vi "Input Entry Init.vi"(8 "Input Control":T2, 9 "Project In":refnum<class "Project.lvclass">, 11 "Refnums":T1) -> (3 "Input Control out":refnum<vi>)   [LabVIEW 2015, in "CallVIStep.lvclass"]
uses:
  CallVIStep.lvclass
  VI Input Control Typedef.ctl
  VI Input Type Typedef.ctl
  Project.lvclass
  <vilib>/Utility/miscctls.llb/LVPointTypeDef.ctl
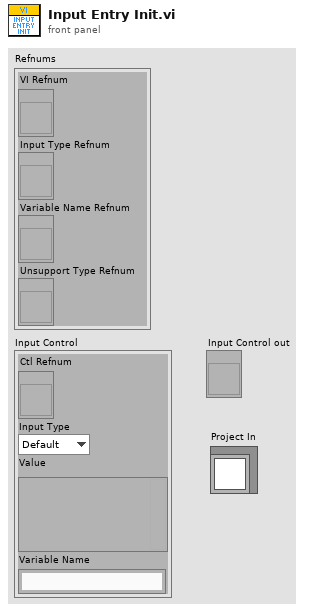
[diagram p1: front panel]
types:
  T1 = cluster{"VI Refnum":refnum<vi>, "Input Type Refnum":refnum<vi>, "Variable Name Refnum":refnum<vi>, "Unsupport Type Refnum":refnum<vi>}
  T2 = typedef "CallVIStep.lvclass/VI Input Control Typedef.ctl" = cluster{"Ctl Refnum":refnum<vi>, "Input Type":T3, "Value":variant, "Variable Name":string}
  T3 = typedef "CallVIStep.lvclass/VI Input Type Typedef.ctl" = enum16{"Default", "Value", "Variable"}
  T4 = enum8{"Enabled", "Disabled", "Disabled and Grayed Out"}
  T5 = typedef "LVPointTypeDef.ctl" = cluster{"Horizontal":i16, "Vertical":i16}
  T6 = typedef "LVBrowseOptionsTypeDef.ctl" = cluster{"Prompt":string, "Match Pattern":string, "select mode":enum32{"existing file", "new file", "new or existing file", "existing dir", "new dir", "new or existing dir", "existing file (use LLBs)", "new file (use LLBs)", "new or existing file (use LLBs)", "new or existing file or directory (use LLBs)", "existing dir (use LLBs)", "new dir (use LLBs)", "new or existing dir (use LLBs)", "existing file or dir", "new file or dir", "new or existing file or dir", "existing file or dir (use LLBs)", "new file or dir (use LLBs)"}, "Start Path":path, "Pattern Label":string, "Button Text":string}
  T7 = typedef "LVComboBoxStrsAndValuesArrayTypeDef.ctl" = cluster{"String":string, "Value":string}[]
  T8 = typedef "LVStringsAndValuesArrayTypeDef.ctl" = cluster{"String":string, "Value":ext}[]
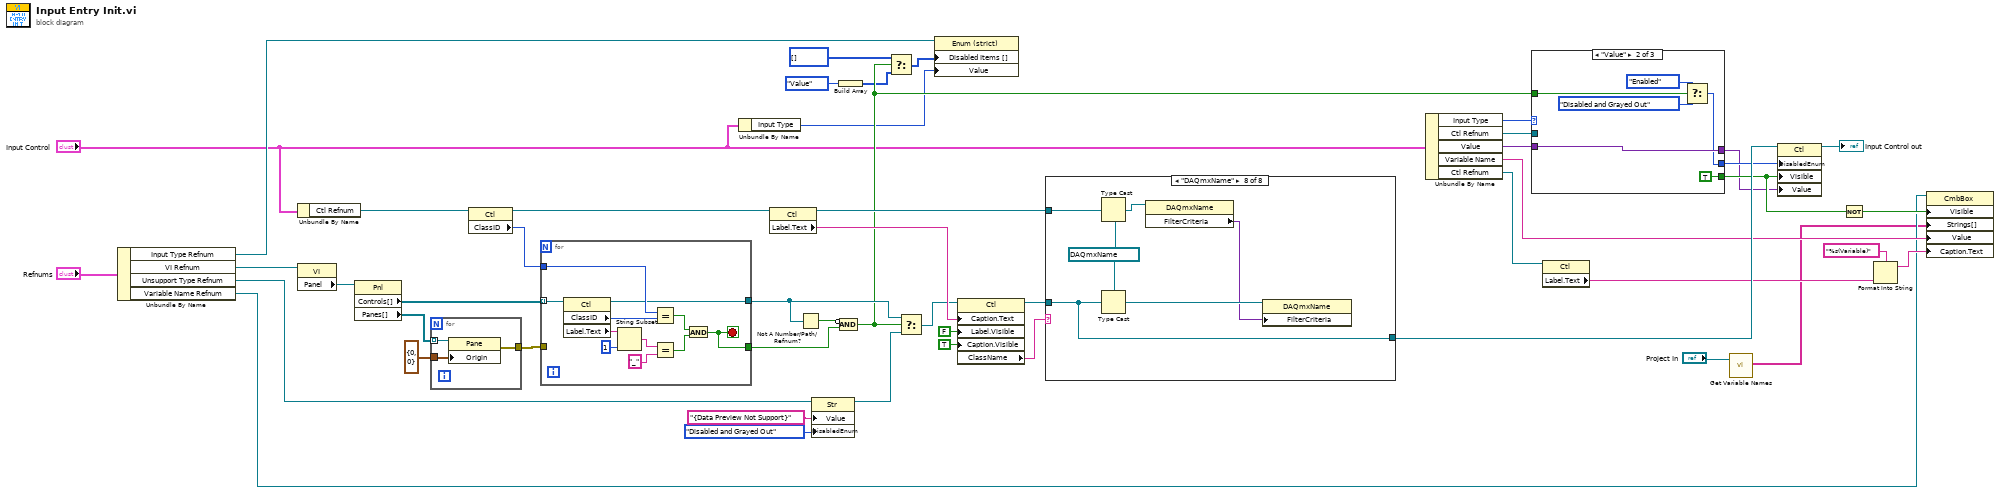
[diagram p0: block diagram]
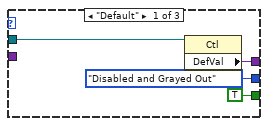
[diagram p2: hidden frame]
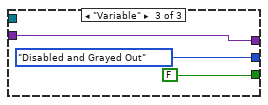
[diagram p3: hidden frame]
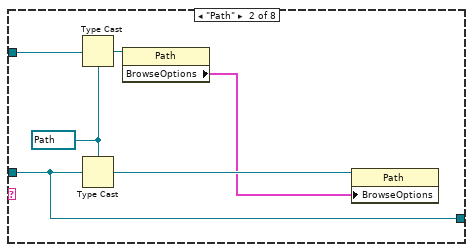
[diagram p5: hidden frame]
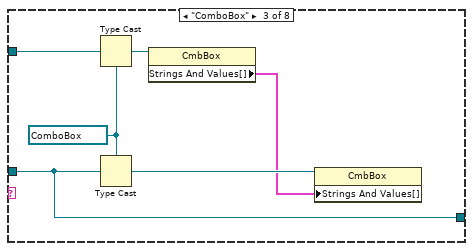
[diagram p6: hidden frame]
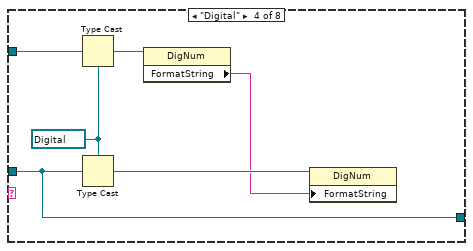
[diagram p7: hidden frame]
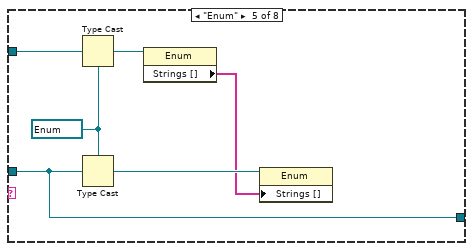
[diagram p8: hidden frame]
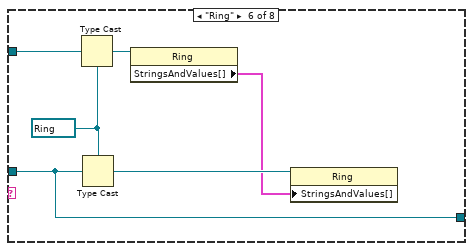
[diagram p9: hidden frame]
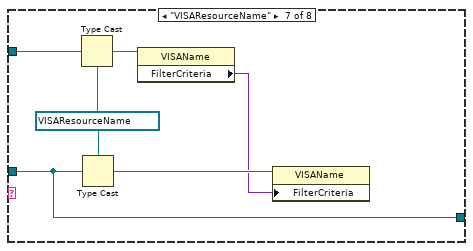
[diagram p10: hidden frame]
diagram:
  n1 = Unbundle By Name("Refnums") -> ("Input Type Refnum"=w6:refnum<vi>, "VI Refnum"=w13:refnum<vi>, "Unsupport Type Refnum"=w12:refnum<vi>, "Variable Name Refnum"=w5:refnum<vi>)
  n2 = Unbundle By Name("Input Control") -> ("Ctl Refnum"=w34:refnum<vi>)
  n3 = property class="VI"(reference=w13) -> ("Panel"=w47:refnum<vi>)  [unwired: 1 in, 2 out]
  n4 = property class="Pnl"(reference=w47) -> ("Controls[]"=w46:refnum<vi>[], "Panes[]"=w49:refnum<vi>[])  [unwired: 1 in, 2 out]
  n5 = for {
    tunnel: w49 -> [w52] mode=indexing
    tunnel: T5 {"Horizontal"=0, "Vertical"=0} ("Origin") -> [w51]
    tunnel: [w50] -> w45
    n6 = property class="Pane"(reference=w52, "Origin"=w51) -> (error out=w50:errorcluster)  [unwired: 1 in, 1 out]
  }
  n7 = property class="Ctl"(reference=w34) -> (reference out=w43:refnum<vi>, "ClassID"=w44:u32)  [unwired: 1 in, 1 out]
  n8 = for {
    tunnel: w46 -> [w63] mode=indexing
    tunnel: w45 -> [_]
    tunnel: w44 -> [w61]
    tunnel: [w54] -> w22
    tunnel: [w53] -> w23
    stop <- w53 stop-if-true
    n9 = property class="Ctl"(reference=w63) -> (reference out=w54:refnum<vi>, "ClassID"=w62:u32, "Label.Text"=w60:string)  [unwired: 1 in, 1 out]
    n10 = String Subset(string=w60, length (rest)=1 ("length (rest)")) -> (substring=w58:string)  [unwired: 1 in]
    n11 = Equal?(x=w61, y=w62) -> (x = y?=w55:bool)
    n12 = Equal?(x=w58, y="_") -> (x = y?=w56:bool)
    n13 = And(x=w55, y=w56) -> (x .and. y?=w53:bool)
  }
  n14 = Unbundle By Name("Input Control") -> ("Input Type"=w3:T3)
  n15 = property class="Ctl"(reference=w43) -> (reference out=w36:refnum<vi>, "Label.Text"=w39:string)  [unwired: 1 in, 1 out]
  n16 = Not A Number/Path/Refnum?(number/path/refnum=w22) -> (NaN/Path/Refnum?=w24:bool)
  n17 = property class="Str"(reference=w12, "Value"="{Data Preview Not Support}", "DisabledEnum"=T4."Disabled and Grayed Out" ("Disabled")) -> (reference out=w20:refnum<vi>)  [unwired: 1 in, 1 out]
  n18 = Build Array(VI_Input_Type_Typedef."Value" ("Input Type")) -> (w7:T3[])
  n19 = Compound Arithmetic op=AND(invert w24, w23) -> (w9:bool)
  n20 = Select(t=i32[] [] ("Disabled Items []"), s=w9, f=w7) -> (s? t:f=w10:i32[])
  n21 = Select(t=w22, s=w9, f=w20) -> (s? t:f=w21:refnum<vi>)
  n22 = property class="Enum (strict)"(reference=w6, "Disabled Items []"=w10, "Value"=w3) -> ()  [unwired: 1 in, 2 out]
  n23 = property class="Ctl"(reference=w21, "Caption.Text"=w39, "Label.Visible"=FALSE, "Caption.Visible"=TRUE) -> (reference out=w37:refnum<vi>, "ClassName"=w38:string)  [unwired: 1 in, 1 out]
  n24 = case shown="\"DAQmxName\"" w38 {
    tunnel: w37 -> [w64 w65 w71 w77 w83 w89 w95 w101]
    tunnel: w36 -> [_ w69 w75 w81 w87 w93 w100 w105]
    tunnel: [w64 w65 w71 w77 w83 w89 w95 w101] -> w35
    frame Default {
    }
    frame "Path" {
      w68 = refnum<vi> refnum ("String in")
      n25 = Type Cast(type=w68, x=w69) -> (*(type *) &x=w67:refnum<vi>)
      n26 = Type Cast(type=w68, x=w65) -> (*(type *) &x=w70:refnum<vi>)
      n27 = property class="Path"(reference=w67) -> ("BrowseOptions"=w66:T6)  [unwired: 1 in, 2 out]
      n28 = property class="Path"(reference=w70, "BrowseOptions"=w66) -> ()  [unwired: 1 in, 2 out]
    }
    frame "ComboBox" {
      w74 = refnum<vi> refnum ("String in")
      n29 = Type Cast(type=w74, x=w75) -> (*(type *) &x=w73:refnum<vi>)
      n30 = Type Cast(type=w74, x=w71) -> (*(type *) &x=w76:refnum<vi>)
      n31 = property class="CmbBox"(reference=w73) -> ("Strings And Values[]"=w72:T7)  [unwired: 1 in, 2 out]
      n32 = property class="CmbBox"(reference=w76, "Strings And Values[]"=w72) -> ()  [unwired: 1 in, 2 out]
    }
    frame "Digital" {
      w80 = refnum<vi> refnum ("String in")
      n33 = Type Cast(type=w80, x=w81) -> (*(type *) &x=w79:refnum<vi>)
      n34 = Type Cast(type=w80, x=w77) -> (*(type *) &x=w82:refnum<vi>)
      n35 = property class="DigNum"(reference=w79) -> ("FormatString"=w78:string)  [unwired: 1 in, 2 out]
      n36 = property class="DigNum"(reference=w82, "FormatString"=w78) -> ()  [unwired: 1 in, 2 out]
    }
    frame "Enum" {
      w86 = refnum<vi> refnum ("String in")
      n37 = Type Cast(type=w86, x=w87) -> (*(type *) &x=w85:refnum<vi>)
      n38 = Type Cast(type=w86, x=w83) -> (*(type *) &x=w88:refnum<vi>)
      n39 = property class="Enum"(reference=w85) -> ("Strings []"=w84:string[])  [unwired: 1 in, 2 out]
      n40 = property class="Enum"(reference=w88, "Strings []"=w84) -> ()  [unwired: 1 in, 2 out]
    }
    frame "Ring" {
      w92 = refnum<vi> refnum ("String in")
      n41 = Type Cast(type=w92, x=w93) -> (*(type *) &x=w91:refnum<vi>)
      n42 = Type Cast(type=w92, x=w89) -> (*(type *) &x=w94:refnum<vi>)
      n43 = property class="Ring"(reference=w91) -> ("StringsAndValues[]"=w90:T8)  [unwired: 1 in, 2 out]
      n44 = property class="Ring"(reference=w94, "StringsAndValues[]"=w90) -> ()  [unwired: 1 in, 2 out]
    }
    frame "VISAResourceName" {
      w99 = refnum<vi> refnum ("String in")
      n45 = Type Cast(type=w99, x=w100) -> (*(type *) &x=w98:refnum<vi>)
      n46 = Type Cast(type=w99, x=w95) -> (*(type *) &x=w97:refnum<vi>)
      n47 = property class="VISAName"(reference=w98) -> ("FilterCriteria"=w96:variant)  [unwired: 1 in, 2 out]
      n48 = property class="VISAName"(reference=w97, "FilterCriteria"=w96) -> ()  [unwired: 1 in, 2 out]
    }
    frame "DAQmxName" {
      w104 = refnum<vi> refnum ("String in")
      n49 = Type Cast(type=w104, x=w105) -> (*(type *) &x=w103:refnum<vi>)
      n50 = Type Cast(type=w104, x=w101) -> (*(type *) &x=w106:refnum<vi>)
      n51 = property class="DAQmxName"(reference=w103) -> ("FilterCriteria"=w102:variant)  [unwired: 1 in, 2 out]
      n52 = property class="DAQmxName"(reference=w106, "FilterCriteria"=w102) -> ()  [unwired: 1 in, 2 out]
    }
  }
  n53 = Unbundle By Name("Input Control") -> ("Input Type"=w31:T3, "Ctl Refnum"=w33:refnum<vi>, "Value"=w32:variant, "Variable Name"=w29:string, "Ctl Refnum"=w28:refnum<vi>)
  n54 = case shown="\"Value\"" w31 {
    tunnel: w33 -> [w110 _ _]
    tunnel: w32 -> [_ w116 w119]
    tunnel: [w108 w116 w119] -> w15
    tunnel: [T4."Disabled and Grayed Out" ("Disabled") w111 T4."Disabled and Grayed Out" ("Disabled")] -> w17
    tunnel: [TRUE TRUE FALSE] -> w16
    tunnel: w9 -> [_ w112 _]
    frame "Default" {
      n55 = property class="Ctl"(reference=w110) -> ("DefVal"=w108:variant)  [unwired: 1 in, 2 out]
    }
    frame "Value" {
      n56 = Select(t=T4."Enabled" ("Disabled"), s=w112, f=T4."Disabled and Grayed Out" ("Disabled")) -> (s? t:f=w111:T4)
    }
    frame "Variable" {
    }
  }
  n57 = property class="Ctl"(reference=w28) -> ("Label.Text"=w26:string)  [unwired: 1 in, 2 out]
  n58 = call "Get Variable Names.vi"("Project in"="Project In") -> ("Variable Names"=w1:string[])  [unwired: 8 in, 2 out]
  n59 = property class="Ctl"(reference=w35, "DisabledEnum"=w17, "Visible"=w16, "Value"=w15) -> (reference out=→"Input Control out":refnum<vi>)  [unwired: 1 in, 1 out]
  n60 = Not(x=w16) -> (.not. x?=w30:bool)
  n61 = Format Into String(format string="%s(Variable)", w26) -> (resulting string=w25:string)  [unwired: 2 in, 1 out]
  n62 = property class="CmbBox"(reference=w5, "Visible"=w30, "Strings[]"=w1, "Value"=w29, "Caption.Text"=w25) -> ()  [unwired: 1 in, 2 out]
